vi "Sonde Measurement Array to Cluster.vi"(10 "Measurements In":dbl[](array[numeric])) -> (2 "Battery Voltage (V)":dbl, 3 "Sonde Data Cluster":T1 caption="Cluster")   [LabVIEW 2016]
uses:
  activeXtest/activeXtest 2015 Folder/sonde cluster.ctl
panel:
  in  "Cluster":T1
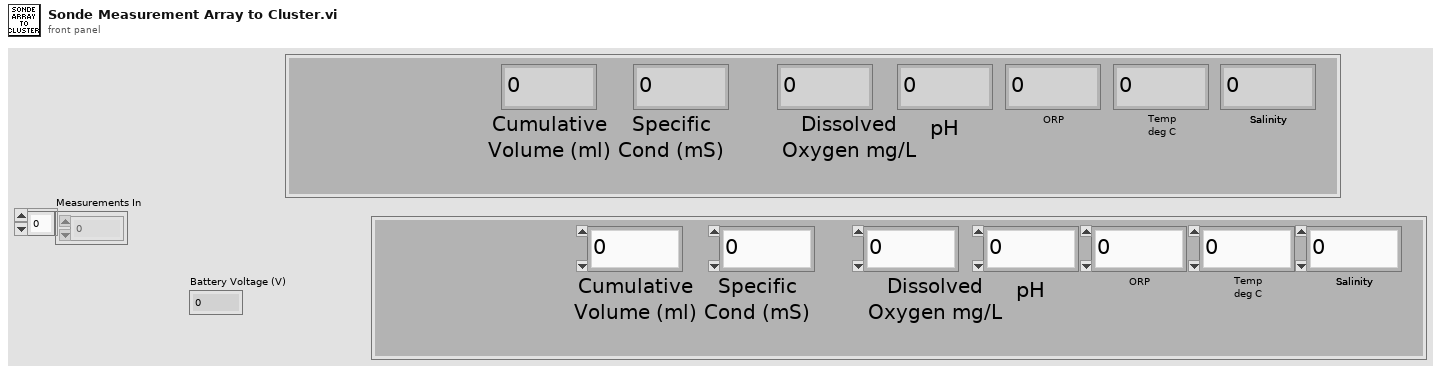
[diagram p1: front panel]
types:
  T1 = typedef "sonde cluster.ctl" = cluster{"Cumulative\nVolume (ml)":dbl, "Specific\nCond (mS)":dbl, "Dissolved\nOxygen mg/L":dbl, "pH":dbl, "ORP":dbl, "Temp\ndeg C":dbl, "Salinity":dbl}
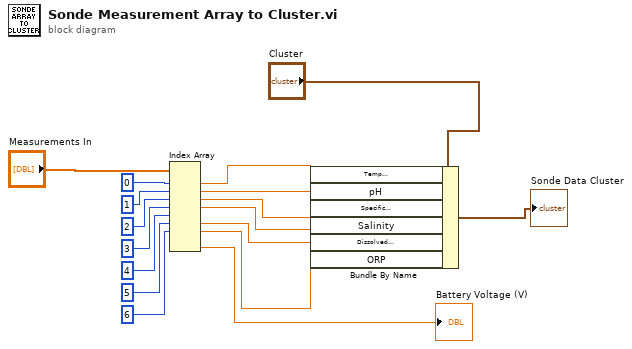
[diagram p0: block diagram]
diagram:
  n1 = Index Array(array="Measurements In", index #1=0 ("index"), index #2=1 ("index"), index #3=2 ("index"), index #4=3 ("index"), index #5=4 ("index"), index #6=5 ("index"), index #7=6 ("index")) -> (element #1=w4:dbl, element #2=w8:dbl, element #3=w9:dbl, element #4=w14:dbl, element #6=w15:dbl, element #7=w16:dbl, element #9=→"Battery Voltage (V)":dbl)  [unwired: 2 in, 2 out]
  n2 = Bundle By Name(cluster="Cluster", "Temp\ndeg C"=w4, "pH"=w8, "Specific\nCond (mS)"=w9, "Salinity"=w14, "Dissolved\nOxygen mg/L"=w15, "ORP"=w16) -> (→"Sonde Data Cluster":T1)
